vi "Read first pulse delay mode.vi"(8 "error in (no error)":errorcluster, 11 "rqcBob in":refnum<class "rqcBob.lvclass">) -> (0 "error out":errorcluster, 2 "rqcBob Pulse Train.First Pulse Delay Mode":T1, 3 "rqcBob out":refnum<class "rqcBob.lvclass">)   [LabVIEW 2019, in "rqcBob.lvclass"]
uses:
  rqcBob.lvclass
  FPGA/rqcBob/Custom Controls/Pulse Train/rqcBob Pulse Train.First Pulse Delay Mode.ctl
  rqcBob.lvclass/rqcBob.ctl
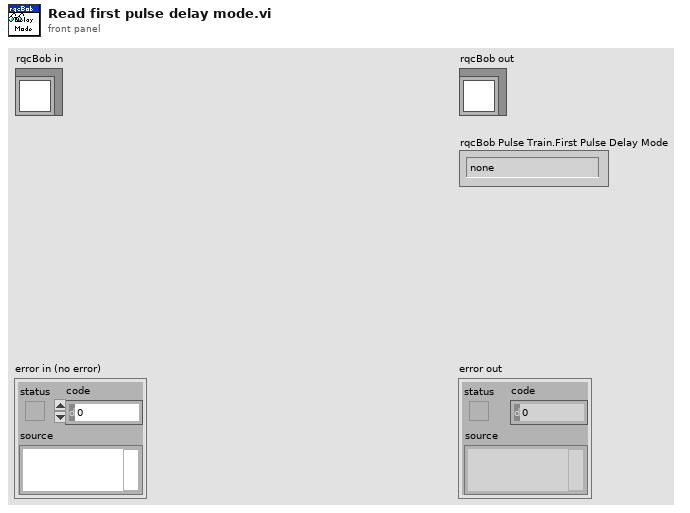
[diagram p1: front panel]
types:
  T1 = typedef "rqcBob Pulse Train.First Pulse Delay Mode.ctl" = enum8{"none", "every train", "first train"}
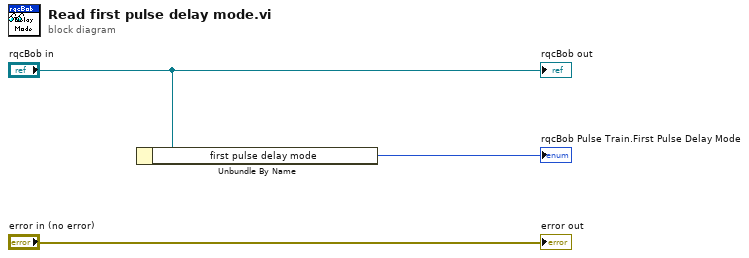
[diagram p0: block diagram]
diagram:
  n1 = Unbundle By Name("rqcBob in") -> ("first pulse delay mode"=→"rqcBob Pulse Train.First Pulse Delay Mode":T1)
  "error out" <- "error in (no error)"
  "rqcBob out" <- "rqcBob in"
